vi "calc_length.vi"(7 "Old length":dbl, 10 "Current point":cluster{"X":i32, "Y":i32}, 11 "Last point":cluster{"X":i32, "Y":i32}) -> (3 "New length":dbl)   [LabVIEW 2011]
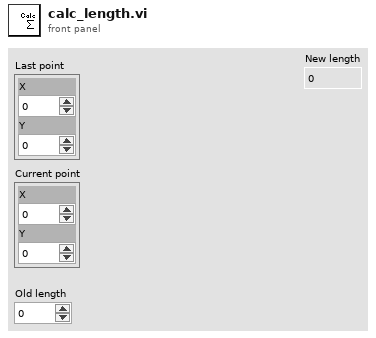
[diagram p1: front panel]
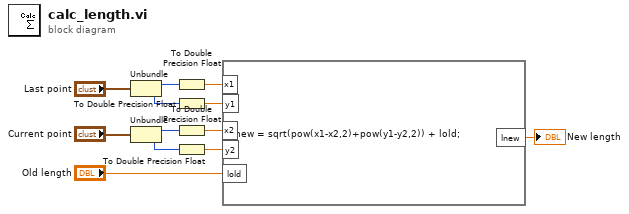
[diagram p0: block diagram]
diagram:
  n1 = Unbundle("Last point") -> ("X"=w8:i32, "Y"=w6:i32)
  n2 = Unbundle("Current point") -> ("X"=w4:i32, "Y"=w2:i32)
  n3 = To Double Precision Float(number=w8) -> (double precision float=w7:dbl)
  n4 = To Double Precision Float(number=w6) -> (double precision float=w5:dbl)
  n5 = To Double Precision Float(number=w4) -> (double precision float=w3:dbl)
  n6 = To Double Precision Float(number=w2) -> (double precision float=w1:dbl)
  n7 = formula code="lnew = sqrt(pow(x1-x2,2)+pow(y1-y2,2)) + lold;"("x1"=w7, "y1"=w5, "x2"=w3, "y2"=w1, "lold"="Old length") -> ("lnew"=→"New length":dbl)
